vi "SetAttributeViBoolean_SE_SpE_Trigger_OB.vi"(7 "AttributeValue (Off)":bool, 8 "error in (no error)":errorcluster {"code" format="%.0x"}, 9 "AttributeID":u32(ring)=1190388 items=["OCCUPIED_BANDWIDTH_AVERAGE_ENABLED"=1190388, "OCCUPIED_BANDWIDTH_DETECTOR_AUTO_ENABLED"=1150069, "OCCUPIED_BANDWIDTH_DISPLAY_WINDOWY_AUTO_SCALE_ENABLED"=1190393, "OCCUPIED_BANDWIDTH_DISPLAY_XDB_BOUNDARIES_ENABLED"=1191464, "OCCUPIED_BANDWIDTH_IF_GAIN"=1190382, "OCCUPIED_BANDWIDTH_IF_GAIN_AUTO_ENABLED"=1190383, "OCCUPIED_BANDWIDTH_LIMIT_TEST_ENABLED"=1190381, "OCCUPIED_BANDWIDTH_MARKER_ENABLED"=1190399, "OCCUPIED_BANDWIDTH_MARKER_MAX_HOLD_ENABLED"=1190385, "OCCUPIED_BANDWIDTH_SWEEPCOUPLING_RESOLUTION_BANDWIDTH_AUTO_ENABLED"=1190410, "OCCUPIED_BANDWIDTH_SWEEPCOUPLING_SWEEP_TIME_AUTO_ENABLED"=1190413, "OCCUPIED_BANDWIDTH_SWEEPCOUPLING_VIDEO_BANDWIDTH_AUTO_ENABLED"=1190415, "SEMASK_AVERAGE_ENABLED"=1190476, "SEMASK_DISPLAY_LIMIT_LINE_ENABLED"=1190490, "SEMASK_DISPLAY_WINDOWX_AUTO_SCALE_ENABLED"=1191465, "SEMASK_DISPLAY_WINDOWY_AUTO_SCALE_ENABLED"=1190489, "SEMASK_MARKER_COUPLE_ENABLED"=1150111, "SEMASK_MARKER_ENABLED"=1190496, "SEMASK_OFFSET_DETECTOR_AUTO_ENABLED"=1150124, "SEMASK_OFFSET_FILTER_ENABLED"=1190499, "SEMASK_REFERENCE_CHANNEL_DETECTOR_AUTO_ENABLED"=1150123, "SEMASK_REFERENCE_CHANNEL_SWEEP_TYPE_AUTO_ENABLED"=1191473, "SEMASK_REFERENCE_CHANNEL_TOTAL_POWER_AUTO_ENABLED"=1190482, "SEMASK_SWEEPCOUPLING_BANDWIDTH_RATIO_AUTO_ENABLED"=1150119, "SEMASK_SWEEPCOUPLING_RESOLUTION_BANDWIDTH_AUTO_ENABLED"=1190480, "SEMASK_SWEEPCOUPLING_SWEEP_TIME_AUTO_ENABLED"=1190484, "SEMASK_SWEEPCOUPLING_VIDEO_BANDWIDTH_AUTO_ENABLED"=1150121, "SIMULATE"=1050005, "SPURIOUS_EMISSIONS_AVERAGE_ENABLED"=1190517, "SPURIOUS_EMISSIONS_DISPLAY_WINDOWY_AUTO_SCALE_ENABLED"=1190522, "SPURIOUS_EMISSIONS_MARKER_COUPLE_ENABLED"=1190526, "SPURIOUS_EMISSIONS_SWEEP_TYPE_AUTO_ENABLED"=1191487, "SPURIOUSEMISSIONS_FAST_MEASUREMENT_ENABLED"=1190665, "SYSTEM_TRACE_ENABLED"=1191770, "TRIGGER_AIQ_MAGNITUDE_DELAY_ENABLED"=1190817, "TRIGGER_AUTO_ENABLED"=1190136, "TRIGGER_EXTERNAL2_DELAY_STATE_ENABLED"=1190143, "TRIGGER_EXTERNAL2_ZERO_SPAN_DELAY_COMPENSATION_ENABLED"=1191483, "TRIGGER_EXTERNAL_DELAY_STATE_ENABLED"=1190139, "TRIGGER_EXTERNAL_ZERO_SPAN_DELAY_COMPENSATION_ENABLED"=1191482, "TRIGGER_FRAME_DELAY_STATE_ENABLED"=1190147, "TRIGGER_FRAME_SYNCHOLDOFF_ENABLED"=1190612, "TRIGGER_HOLDOFF_ENABLED"=1190156, "TRIGGER_I_DEMODULATED_DELAY_ENABLED"=1190821, "TRIGGER_INPUT_I_DELAY_ENABLED"=1190825, "TRIGGER_INPUT_Q_DELAY_ENABLED"=1190837, "TRIGGER_IQ_MAGNITUDE_DELAY_ENABLED"=1190829, "TRIGGER_LINE_DELAY_STATE_ENABLED"=1190159, "TRIGGER_Q_DEMODULATED_DELAY_ENABLED"=1190833, "TRIGGER_RFBURST_DELAY_STATE_ENABLED"=1190162, "TRIGGER_SWEEP_MODE_CONTINUOUS_ENABLED"=1190581, "TRIGGER_VIDEO_DELAY_STATE_ENABLED"=1190168, "TYPE_AUTO_ENABLED"=1191710], 10 "RepCapIdentifier":string, 11 "instrument handle":refnum<k15>) -> (0 "error out":errorcluster {"code" format="%.0x"}, 3 "instrument handle out":refnum<k15>)   [LabVIEW 2021, in "Keysight XSAnVMA.lvlib"]
doc: "Sets Boolean Attribute from instrumrnt driver.\nThe following attributes are supported:\n\nOCCUPIED_BANDWIDTH_AVERAGE_ENABLED\nOCCUPIED_BANDWIDTH_DETECTOR_AUTO_ENABLED\nOCCUPIED_BANDWIDTH_DISPLAY_WINDOWY_AUTO_SCALE_ENABLED\nOCCUPIED_BANDWIDTH_DISPLAY_XDB_BOUNDARIES_ENABLED\nOCCUPIED_BANDWIDTH_IF_GAIN\nOCCUPIED_BANDWIDTH_IF_GAIN_AUTO_ENABLED\nOCCUPIED_BANDWIDTH_LIMIT_TEST_ENABLED\nOCCUPIED_BANDWIDTH_MARKER_ENABLED\nOCCUPIED_BANDWIDTH_MARKER_MAX_HOLD_ENABLED\nOCCUPIED_BANDWIDTH_SWEEPCOUPLING_RESOLUTION_BANDWIDTH_AUTO_ENABLED\nOCCUPIED_BANDWIDTH_SWEEPCOUPLING_SWEEP_TIME_AUTO_ENABLED\nOCCUPIED_BANDWIDTH_SWEEPCOUPLING_VIDEO_BANDWIDTH_AUTO_ENABLED\nSEMASK_AVERAGE_ENABLED\nSEMASK_DISPLAY_LIMIT_LINE_ENABLED\nSEMASK_DISPLAY_WINDOWX_AUTO_SCALE_ENABLED\nSEMASK_DISPLAY_WINDOWY_AUTO_SCALE_ENABLED\nSEMASK_MARKER_COUPLE_ENABLED\nSEMASK_MARKER_ENABLED\nSEMASK_OFFSET_DETECTOR_AUTO_ENABLED\nSEMASK_OFFSET_FILTER_ENABLED\nSEMASK_REFERENCE_CHANNEL_DETECTOR_AUTO_ENABLED\nSEMASK_REFERENCE_CHANNEL_SWEEP_TYPE_AUTO_ENABLED\nSEMASK_REFERENCE_CHANNEL_TOTAL_POWER_AUTO_ENABLED\nSEMASK_SWEEPCOUPLING_BANDWIDTH_RATIO_AUTO_ENABLED\nSEMASK_SWEEPCOUPLING_RESOLUTION_BANDWIDTH_AUTO_ENABLED\nSEMASK_SWEEPCOUPLING_SWEEP_TIME_AUTO_ENABLED\nSEMASK_SWEEPCOUPLING_VIDEO_BANDWIDTH_AUTO_ENABLED\nSIMULATE\nSPURIOUS_EMISSIONS_AVERAGE_ENABLED\nSPURIOUS_EMISSIONS_DISPLAY_WINDOWY_AUTO_SCALE_ENABLED\nSPURIOUS_EMISSIONS_MARKER_COUPLE_ENABLED\nSPURIOUS_EMISSIONS_SWEEP_TYPE_AUTO_ENABLED\nSPURIOUSEMISSIONS_FAST_MEASUREMENT_ENABLED\nSYSTEM_TRACE_ENABLED\nTRIGGER_AIQ_MAGNITUDE_DELAY_ENABLED\nTRIGGER_AUTO_ENABLED\nTRIGGER_EXTERNAL2_DELAY_STATE_ENABLED\nTRIGGER_EXTERNAL2_ZERO_SPAN_DELAY_COMPENSATION_ENABLED\nTRIGGER_EXTERNAL_DELAY_STATE_ENABLED\nTRIGGER_EXTERNAL_ZERO_SPAN_DELAY_COMPENSATION_ENABLED\nTRIGGER_FRAME_DELAY_STATE_ENABLED\nTRIGGER_FRAME_SYNCHOLDOFF_ENABLED\nTRIGGER_HOLDOFF_ENABLED\nTRIGGER_I_DEMODULATED_DELAY_ENABLED\nTRIGGER_INPUT_I_DELAY_ENABLED\nTRIGGER_INPUT_Q_DELAY_ENABLED\nTRIGGER_IQ_MAGNITUDE_DELAY_ENABLED\nTRIGGER_LINE_DELAY_STATE_ENABLED\nTRIGGER_Q_DEMODULATED_DELAY_ENABLED\nTRIGGER_RFBURST_DELAY_STATE_ENABLED\nTRIGGER_SWEEP_MODE_CONTINUOUS_ENABLED\nTRIGGER_VIDEO_DELAY_STATE_ENABLED\nTYPE_AUTO_ENABLED"
uses:
  <instrlib>/Keysight XSAnVMA/Keysight XSAnVMA.lvlib
  KtXSAnVMA_64.dll
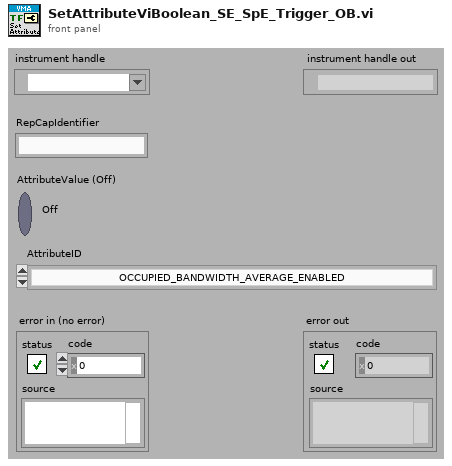
[diagram p1: front panel]
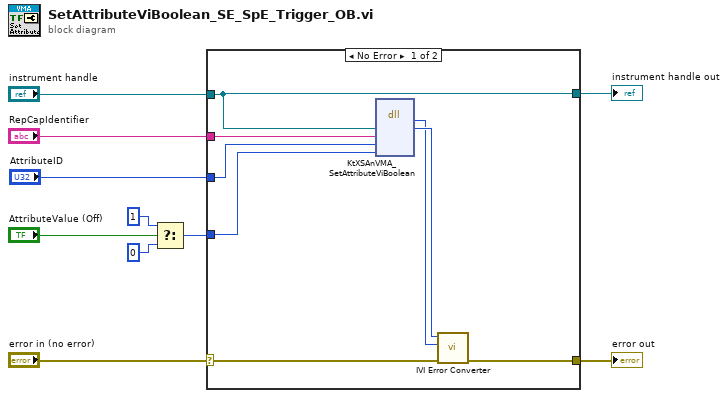
[diagram p0: block diagram]
diagram:
  n1 = Select(t=u16 1, s="AttributeValue (Off)", f=u16 0) -> (s? t:f=w3:u16)
  n2 = case shown="No Error" "error in (no error)" {
    selector: "error in (no error)" -> [w16 w20]
    tunnel: [w15 w20] -> w10
    tunnel: "instrument handle" -> [w11 w19]
    tunnel: "RepCapIdentifier" -> [w14 _]
    tunnel: "AttributeID" -> [w13 _]
    tunnel: w3 -> [w12 _]
    tunnel: [w11 w19] -> w2
    frame No Error {
      n3 = dll-call lib="KtXSAnVMA**.dll" fn="KtXSAnVMA_SetAttributeViBoolean"("Vi"=w11, "RepCapIdentifier"=w14, "AttributeID"=w13, "AttributeValue"=w12) -> ("return type"=w17:i32, "Vi"=w18:u32)  [unwired: 6 in, 2 out]
      n4 = call <instrlib>:"IVI Error Converter.vi"("error in (no error)"=w16, "IVI error code (0)"=w17, "instrument handle"=w18) -> ("error out"=w15:errorcluster)  [unwired: 7 in, 1 out]
    }
    frame Error {
    }
  }
  "error out" <- w10
  "instrument handle out" <- w2
